vi "Top_main.vi"() -> ()   [LabVIEW 2016]
uses:
  <vilib>/Utility/NIReport.llb/NI_report.lvclass
  <vilib>/addons/_office/excel.llb/Excel Easy Table (str).vi
  <vilib>/addons/_office/NI_ReportGenerationToolkit.lvlib
  <vilib>/Utility/NIReport.llb/Excel/NI_Excel.lvclass
panel:
  in  "문자열":string
  out "next cell bottom-left":cluster{"row":i32, "column":i32}
  out "next cell top-right":cluster{"row":i32, "column":i32}
  out "report out":refnum<class "NI_report.lvclass">
  in  "Probe Name":string
  in  "Measure Station Setup":T1 {"scopeResistOhm" format="%.2f"; "scopeCapacityF" format="%.2e"}
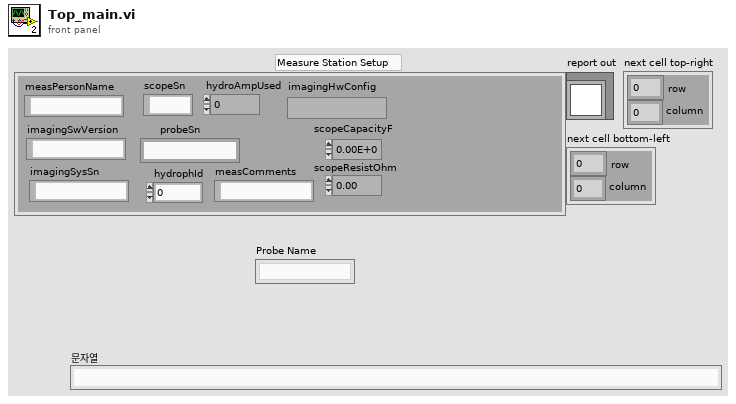
[diagram p1: front panel]
types:
  T1 = cluster{"imagingSwVersion":string, "measPurpose":string, "measComments":string, "probeId":i32, "hydrophId":i16, "probeSn":string, "measPersonName":string, "imagingSysSn":string, "labviewSwVersion":string, "scopeSn":string, "scopeCapacityF":sgl, "scopeResistOhm":sgl, "hydroAmpUsed":i8, "imagingHwConfig":string, "measSSId":i32}
  T2 = enum16{"Standard Report", "HTML", "Word", "Excel"}
  T3 = typedef "Generate Report Object Reference.ctl" = refnum<class "NI_report.lvclass">
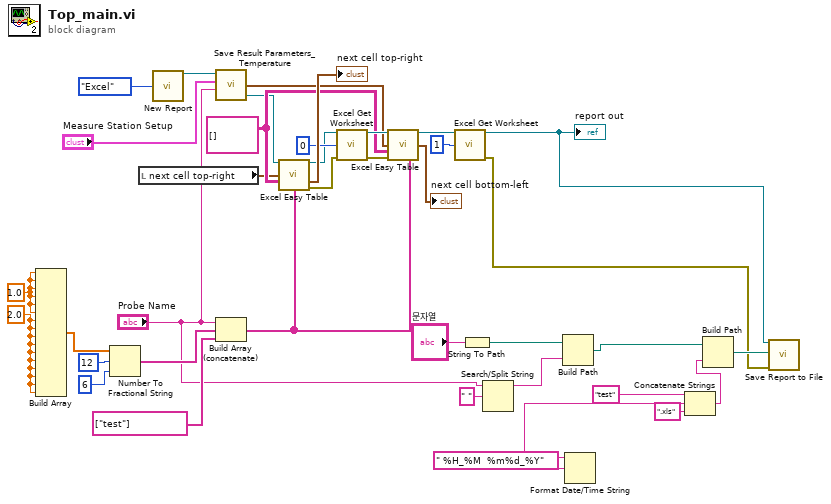
[diagram p0: block diagram]
diagram:
  w15 = 2.0 ("원소")
  w16 = 1.0 ("원소")
  w26 = string[][] [] ("numerical data")
  n1 = Build Array(w16, w16, w16, w16, w16, w16, w15, w15, w15, w15, w15, w15, w15, w15, w15, w15) -> (w33:dbl[])
  n2 = Number To Fractional String(number=w33, width (-)=i16 12, precision (6)=i16 6) -> (F-format string=w32:string[])  [unwired: 1 in]
  n3 = local read "next cell top-right"() -> (w18:cluster{"row":i32, "column":i32})
  n4 = call <vilib>:"New Report.vi"("report type"=T2."Excel") -> ("report out"=w37:refnum<class "NI_report.lvclass">)  [unwired: 13 in, 1 out]
  n5 = call "Save Result Parameters_Temperature.vi"("report In"=w37, "Measure Station Setup"="Measure Station Setup", "Probe Name"="Probe Name") -> ("next cell bottom-left"=w19:cluster{"row":i32, "column":i32}, "report out"=w20:T3)  [unwired: 4 in]
  n6 = Build Array (concatenate)("Probe Name", w32, string[] ["test"] ("원소")) -> (w24:string[])
  n7 = call-poly <vilib>:"Excel Easy Table.vi"("report in"=w20, "start (0, 0)"=w18, "text data"=w26, "row headers"=w24) -> ("report out"=w30:refnum<class "NI_report.lvclass">, "next cell top-right"=→"next cell top-right":cluster{"row":i32, "column":i32}, "error out"=w29:errorcluster)  [unwired: 7 in, 2 out]
  n8 = call <vilib>:"Excel Get Worksheet.vi"("report in"=w30, "worksheet index (0)"=0, "error in (no error)"=w29) -> ("report out"=w28:refnum<class "NI_report.lvclass">, "error out"=w27:errorcluster)  [unwired: 11 in]
  n9 = call-poly <vilib>:"Excel Easy Table.vi"("report in"=w28, "start (0, 0)"=w19, "text data"=w26, "error in (no error)"=w27, "column headers"=w24) -> ("report out"=w23:refnum<class "NI_report.lvclass">, "next cell bottom-left"=→"next cell bottom-left":cluster{"row":i32, "column":i32})  [unwired: 6 in, 3 out]
  n10 = call <vilib>:"Excel Get Worksheet.vi"("report in"=w23, "worksheet index (0)"=1) -> ("report out"=w4:refnum<class "NI_report.lvclass">, "error out"=w2:errorcluster)  [unwired: 12 in]
  "report out" <- w4
  n11 = String To Path(string="문자열") -> (path=w7:path)
  n12 = Search/Split String(string="Probe Name", search string/char (-)=" ") -> (substring before match=w11:string)  [unwired: 1 in, 2 out]
  n13 = Build Path(base path=w7, name or relative path=w11) -> (appended path=w1:path)
  n14 = Format Date/Time String(time format string (%c)=" %H_%M  %m%d_%Y") -> (date/time string=w10:string)  [unwired: 2 in]
  n15 = Concatenate Strings("test" ("문자열"), w10, ".xls" ("string")) -> (w9:string)
  n16 = Build Path(base path=w1, name or relative path=w9) -> (appended path=w3:path)
  n17 = call-dynamic "Save Report to File.vi"("report in"=w4, "report file path"=w3, "error in (no error)"=w2) -> ()  [unwired: 11 in, 2 out]
